vi "VI Tree.vi"   [LabVIEW 2010, in "Tektronix TDS 3000 Series.lvlib"]
doc: "This is the VI Tree for the Tektronix TDS 3xxx series instrument driver. It displays all the VIs of the instrument driver in an organized table."
uses:
  <instrlib>/Tektronix TDS 3000 Series/Tektronix TDS 3000 Series.lvlib
panel:
  # "© 2003-2006, National Instruments, Corporation.  All Rights Reserved."
  # "SEE DIAGRAM\nFOR VI TREE."
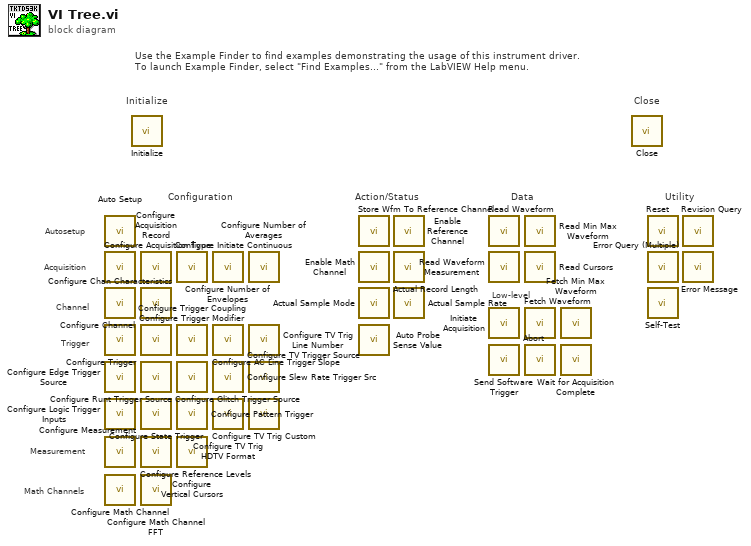
[diagram p0: block diagram]
diagram:
  # "Math Channels"
  # "Measurement"
  # "Trigger"
  # "Channel"
  # "Acquisition"
  # "Autosetup"
  # "Low-level"
  # "Action/Status"
  # "Data"
  # "Use the Example Finder to find examples demonstrating the usage of this instrument driver.\nTo launch Example Finder, select \"Find Examples...\" from the LabVIEW Help menu."
  # "Close"
  # "Utility"
  # "Configuration"
  # "Initialize"
  n1 = call <instrlib>:"Auto Setup.vi"() -> ()  [unwired: 10 in, 2 out]
  n2 = call <instrlib>:"Configure Acquisition Type.vi"() -> ()  [unwired: 10 in, 2 out]
  n3 = call <instrlib>:"Configure Channel.vi"() -> ()  [unwired: 10 in, 2 out]
  n4 = call <instrlib>:"Configure Trigger.vi"() -> ()  [unwired: 10 in, 2 out]
  n5 = call <instrlib>:"Configure Edge Trigger Source.vi"() -> ()  [unwired: 10 in, 2 out]
  n6 = call <instrlib>:"Configure Logic Trigger Inputs.vi"() -> ()  [unwired: 14 in, 2 out]
  n7 = call <instrlib>:"Configure Measurement.vi"() -> ()  [unwired: 10 in, 2 out]
  n8 = call <instrlib>:"Configure Math Channel.vi"() -> ()  [unwired: 10 in, 2 out]
  n9 = call <instrlib>:"Initialize.vi"() -> ()  [unwired: 10 in, 2 out]
  n10 = call <instrlib>:"Configure Acquisition Record.vi"() -> ()  [unwired: 14 in, 2 out]
  n11 = call <instrlib>:"Configure Chan Characteristics.vi"() -> ()  [unwired: 14 in, 2 out]
  n12 = call <instrlib>:"Configure Trigger Modifier.vi"() -> ()  [unwired: 10 in, 2 out]
  n13 = call <instrlib>:"Configure Runt Trigger Source.vi"() -> ()  [unwired: 14 in, 2 out]
  n14 = call <instrlib>:"Configure State Trigger.vi"() -> ()  [unwired: 10 in, 2 out]
  n15 = call <instrlib>:"Configure Reference Levels.vi"() -> ()  [unwired: 14 in, 2 out]
  n16 = call <instrlib>:"Configure Math Channel FFT.vi"() -> ()  [unwired: 10 in, 2 out]
  n17 = call <instrlib>:"Configure Initiate Continuous.vi"() -> ()  [unwired: 10 in, 2 out]
  n18 = call <instrlib>:"Configure Trigger Coupling.vi"() -> ()  [unwired: 10 in, 2 out]
  n19 = call <instrlib>:"Configure Glitch Trigger Source.vi"() -> ()  [unwired: 14 in, 2 out]
  n20 = call <instrlib>:"Configure Pattern Trigger.vi"() -> ()  [unwired: 10 in, 2 out]
  n21 = call <instrlib>:"Configure Vertical Cursors.vi"() -> ()  [unwired: 10 in, 2 out]
  n22 = call <instrlib>:"Configure Number of Envelopes.vi"() -> ()  [unwired: 10 in, 2 out]
  n23 = call <instrlib>:"Configure AC Line Trigger Slope.vi"() -> ()  [unwired: 10 in, 2 out]
  n24 = call <instrlib>:"Configure Slew Rate Trigger Src.vi"() -> ()  [unwired: 14 in, 2 out]
  n25 = call <instrlib>:"Configure TV Trig HDTV Format.vi"() -> ()  [unwired: 10 in, 2 out]
  n26 = call <instrlib>:"Configure Number of Averages.vi"() -> ()  [unwired: 10 in, 2 out]
  n27 = call <instrlib>:"Configure TV Trig Line Number.vi"() -> ()  [unwired: 10 in, 2 out]
  n28 = call <instrlib>:"Configure TV Trigger Source.vi"() -> ()  [unwired: 14 in, 2 out]
  n29 = call <instrlib>:"Configure TV Trig Custom.vi"() -> ()  [unwired: 10 in, 2 out]
  n30 = call <instrlib>:"Store Wfm To Reference Channel.vi"() -> ()  [unwired: 10 in, 2 out]
  n31 = call <instrlib>:"Enable Math Channel.vi"() -> ()  [unwired: 10 in, 2 out]
  n32 = call <instrlib>:"Actual Sample Mode.vi"() -> ()  [unwired: 9 in, 3 out]
  n33 = call <instrlib>:"Auto Probe Sense Value.vi"() -> ()  [unwired: 9 in, 3 out]
  n34 = call <instrlib>:"Enable Reference Channel.vi"() -> ()  [unwired: 10 in, 2 out]
  n35 = call <instrlib>:"Actual Record Length.vi"() -> ()  [unwired: 9 in, 3 out]
  n36 = call <instrlib>:"Actual Sample Rate.vi"() -> ()  [unwired: 9 in, 3 out]
  n37 = call <instrlib>:"Read Waveform.vi"() -> ()  [unwired: 6 in, 6 out]
  n38 = call <instrlib>:"Read Waveform Measurement.vi"() -> ()  [unwired: 9 in, 3 out]
  n39 = call <instrlib>:"Initiate Acquisition.vi"() -> ()  [unwired: 10 in, 2 out]
  n40 = call <instrlib>:"Send Software Trigger.vi"() -> ()  [unwired: 10 in, 2 out]
  n41 = call <instrlib>:"Read Min Max Waveform.vi"() -> ()  [unwired: 5 in, 7 out]
  n42 = call <instrlib>:"Read Cursors.vi"() -> ()  [unwired: 6 in, 10 out]
  n43 = call <instrlib>:"Fetch Waveform.vi"() -> ()  [unwired: 6 in, 6 out]
  n44 = call <instrlib>:"Abort.vi"() -> ()  [unwired: 10 in, 2 out]
  n45 = call <instrlib>:"Fetch Min Max Waveform.vi"() -> ()  [unwired: 5 in, 7 out]
  n46 = call <instrlib>:"Wait for Acquisition Complete.vi"() -> ()  [unwired: 10 in, 2 out]
  n47 = call <instrlib>:"Close.vi"() -> ()  [unwired: 11 in, 1 out]
  n48 = call <instrlib>:"Reset.vi"() -> ()  [unwired: 10 in, 2 out]
  n49 = call <instrlib>:"Error Query (Multiple).vi"() -> ()  [unwired: 8 in, 4 out]
  n50 = call <instrlib>:"Self-Test.vi"() -> ()  [unwired: 8 in, 4 out]
  n51 = call <instrlib>:"Revision Query.vi"() -> ()  [unwired: 12 in, 4 out]
  n52 = call <instrlib>:"Error Message.vi"() -> ()  [unwired: 11 in, 5 out]
